vi "rad_ForceSafeMode.vi"(8 "error in (no error)":errorcluster, 11 "Target in":refnum<k21>) -> (0 "error out":errorcluster, 3 "Target out":refnum<k21>)   [LabVIEW 2023]
uses:
  <vilib>/nisyscfg/Save Changes (Hardware).vi
  <vilib>/nisyscfg/Close (Hardware).vi
  <resource>/objmgr/nisysapi.rc
  <vilib>/nisyscfg/nisyscfg.lvlib
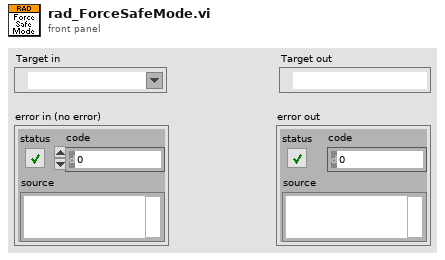
[diagram p1: front panel]
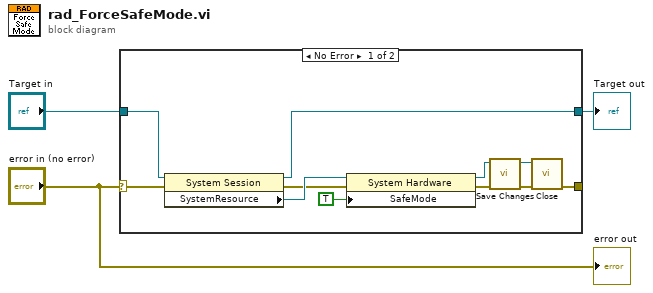
[diagram p0: block diagram]
diagram:
  n1 = case shown="No Error" "error in (no error)" {
    selector: "error in (no error)" -> [w6 w16]
    tunnel: "Target in" -> [w14 w15]
    tunnel: [w5 w16] -> _
    tunnel: [w4 w15] -> w2
    frame No Error {
      n2 = property class="System Session"(reference=w14, error in=w6) -> (reference out=w4:refnum<k21>, error out=w12:errorcluster, "SystemResource"=w13:refnum<k20>)
      n3 = property class="System Hardware"(reference=w13, error in=w12, "SafeMode"=TRUE ("Startup Settings:User Directed Safe Mode")) -> (reference out=w9:refnum<k20>, error out=w10:errorcluster)
      n4 = call-poly <vilib>:"Save Changes.vi"("error in (no error)"=w10, "Resource in"=w9) -> ("error out"=w7:errorcluster, "Resource out"=w8:refnum<k20>)  [unwired: 6 in, 2 out]
      n5 = call-poly <vilib>:"Close.vi"("error in (no error)"=w7, "Resource in"=w8) -> ("error out"=w5:errorcluster)  [unwired: 9 in]
    }
    frame Error {
    }
  }
  "Target out" <- w2
  "error out" <- "error in (no error)"
